vi "Update Run Pause UI State.vi"(7 "Plugin Name":string, 8 "error in (no error)":errorcluster, 10 "Index":i32, 11 "CIF_UI in":refnum<class "CIF_UI.lvclass">) -> (0 "error out":errorcluster, 3 "CIF_UI out":refnum<class "CIF_UI.lvclass">)   [LabVIEW 2021, in "CIF_UI.lvclass"]
uses:
  CIF_UI.lvclass
  CIF_UI.lvclass/CIF_UI.ctl
  CIFCore/Grpc/CIFCoreWrapper/CIFCoreWrapper.lvlib
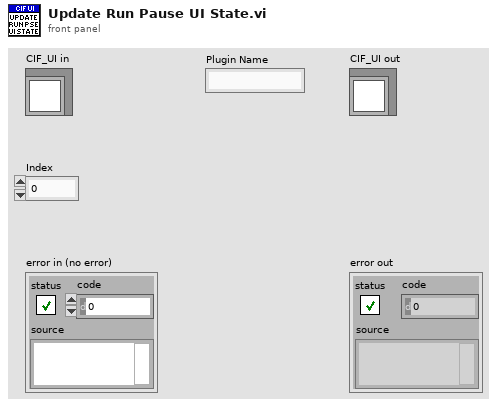
[diagram p1: front panel]
types:
  T1 = typedef "grpc-lvsupport-release.lvlib/grpcId.ctl" = u64
  T2 = typedef "CIFCoreCommon.lvlib/gRPC Reported Plugin Status.ctl" = cluster{"State":T3, "Timing Statistics (us)":T4, "FIFO Statistics (us)":T6, "error":T7, "Monitor Doubles":T8, "Monitor U64":T9, "Monitor I64":T10}
  T3 = typedef "CIFCoreCommon.lvlib/Plugin State.ctl" = enum32{"Null", "Creating", "Listening", "Running", "CleaningUp", "Destroying"}
  T4 = typedef "CIFCoreCommon.lvlib/Timing Statistics.ctl" = cluster{"Period":T5, "Wake Error":T5, "Execute":T5, "Housekeep":T5, "Idle":T5, "Cleanup":T5, "Custom 1 (custom units)":T5, "Custom 2 (custom units)":T5}
  T5 = typedef "CIFCoreCommon.lvlib/Timing Stats Base.ctl" = cluster{"Max":i64, "Avg":dbl, "Min":i64}
  T6 = typedef "CIFCoreCommon.lvlib/FIFO Statistics.ctl" = cluster{"From T0":T5, "From Previous Plugin":T5, "Output Error":T5}
  T7 = typedef "CIFCoreCommon.lvlib/Simple Error.ctl" = cluster{"status":bool, "code":i32}
  T8 = typedef "CIFCoreCommon.lvlib/Monitor Doubles.ctl" = cluster{"1":dbl, "2":dbl, "3":dbl, "4":dbl}
  T9 = typedef "CIFCoreCommon.lvlib/Monitor U64.ctl" = cluster{"1":u64, "2":u64, "3":u64, "4":u64}
  T10 = typedef "CIFCoreCommon.lvlib/Monitor I64.ctl" = cluster{"1":i64, "2":i64, "3":i64, "4":i64}
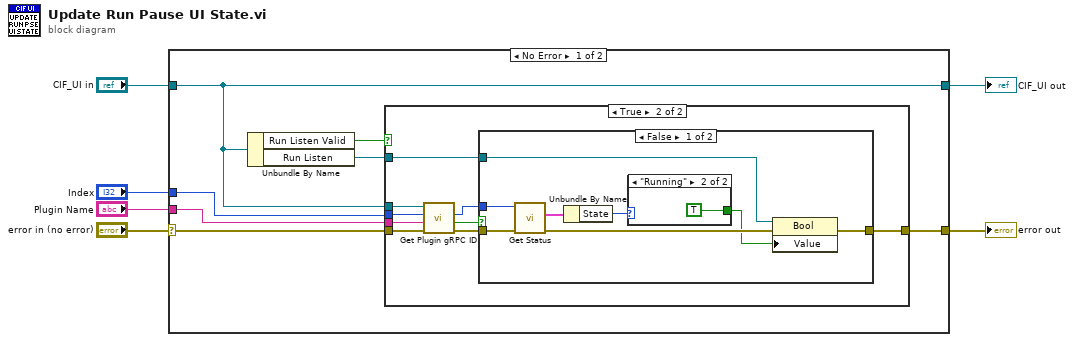
[diagram p0: block diagram]
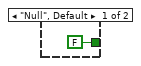
[diagram p3: hidden frame]
diagram:
  n1 = case shown="No Error" "error in (no error)" {
    selector: "error in (no error)" -> [w10 w36]
    tunnel: [w7 w36] -> w5
    tunnel: [w11 w35] -> w3
    tunnel: "CIF_UI in" -> [w11 w35]
    tunnel: "Plugin Name" -> [w9 _]
    tunnel: "Index" -> [w8 _]
    frame No Error {
      n2 = Unbundle By Name(w11) -> ("Run Listen Valid"=w13:bool, "Run Listen"=w12:refnum<vi>)
      n3 = case shown="True" w13 {
        tunnel: w12 -> [_ w16]
        tunnel: w11 -> [_ w20]
        tunnel: w10 -> [w14 w17]
        tunnel: w9 -> [_ w19]
        tunnel: w8 -> [_ w18]
        tunnel: [w14 w15] -> w7
        frame False {
        }
        frame True {
          n4 = call "Get Plugin gRPC ID.vi"("error in (no error)"=w17, "Plugin Name"=w19, "Index"=w18, "CIF_UI in"=w20) -> ("error out"=w21:errorcluster, "Not Found"=w22:bool, "gRPC ID"=w23:T1)  [unwired: 4 in, 1 out]
          n5 = case shown="False" w22 {
            tunnel: w23 -> [w31 _]
            tunnel: w21 -> [w30 w34]
            tunnel: [w27 w34] -> w15
            tunnel: w16 -> [w29 _]
            frame False {
              n6 = call "Get Status.vi"("error in"=w30, "gRPC ID"=w31) -> ("error out"=w28:errorcluster, "Node Status"=w26:T2)  [unwired: 7 in, 1 out]
              n7 = Unbundle By Name(w26) -> ("State"=w25:T3)
              n8 = case shown="\"Running\"" w25 {
                tunnel: [FALSE TRUE] -> w24
                frame "Null", Default {
                }
                frame "Running" {
                }
              }
              n9 = property class="Bool"(reference=w29, error in=w28, "Value"=w24) -> (error out=w27:errorcluster)  [unwired: 1 out]
            }
            frame True {
            }
          }
        }
      }
    }
    frame Error {
    }
  }
  "error out" <- w5
  "CIF_UI out" <- w3
